vi "登陆界面.vi"() -> ()   [LabVIEW 2014]
panel:
  in  "注册":bool
  in  "游客登陆":bool
  out "学号与姓名表路径":path
  out "tips":string
  in  "姓  名":string
  in  "学  号":string
  in  "退出":bool
  in  "登陆":bool
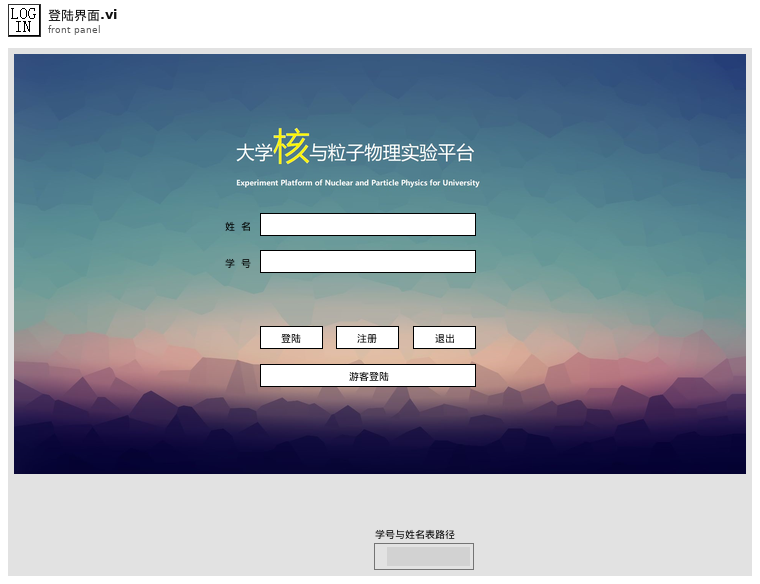
[diagram p1: front panel]
types:
  T1 = typedef "枚举常量_登陆界面.ctl" = enum16{"初始化", "等待用户输入", "信息匹配", "退出"}
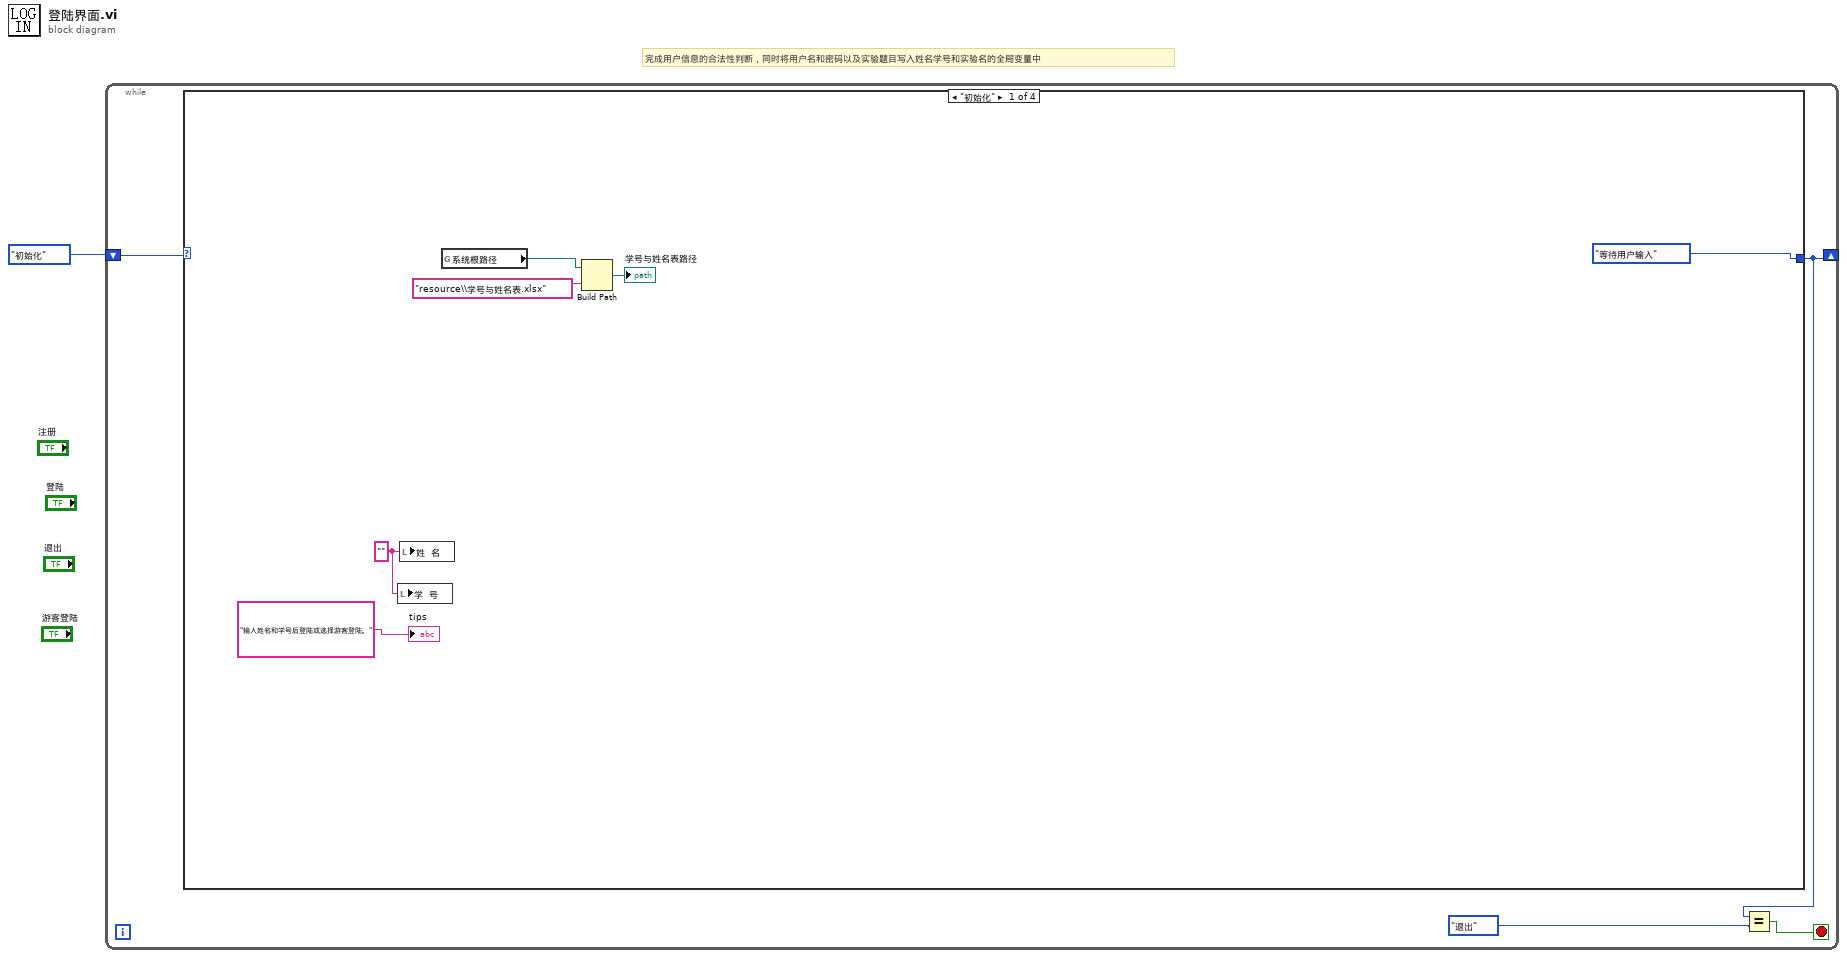
[diagram p0: block diagram]
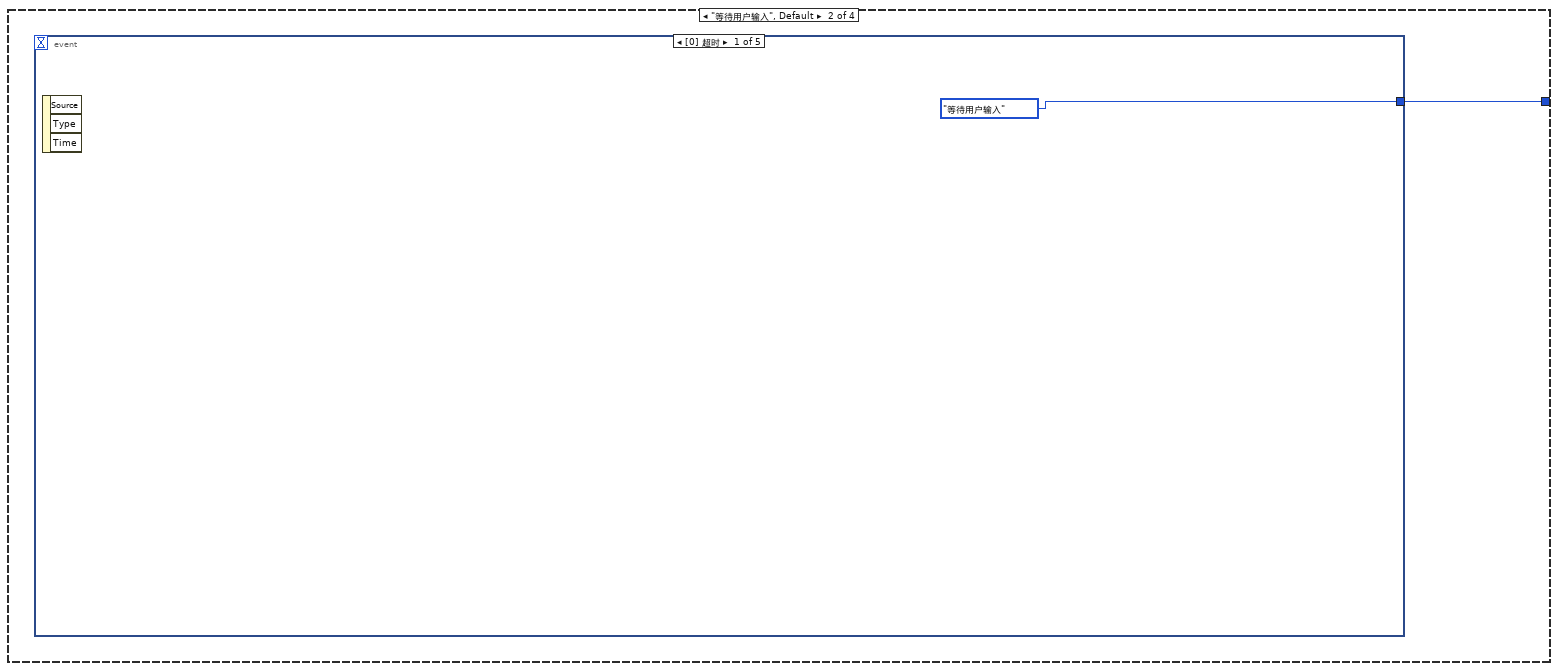
[diagram p2: hidden frame]
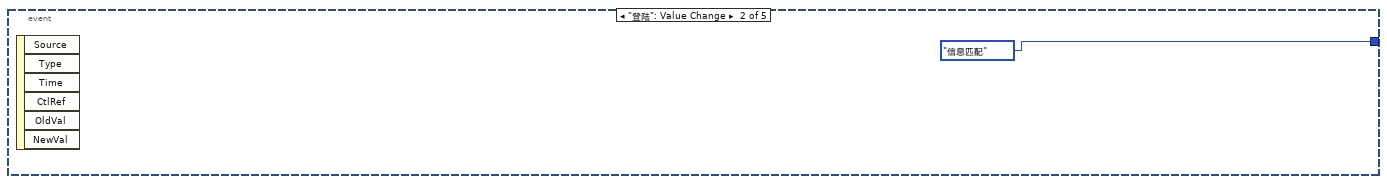
[diagram p3: hidden frame]
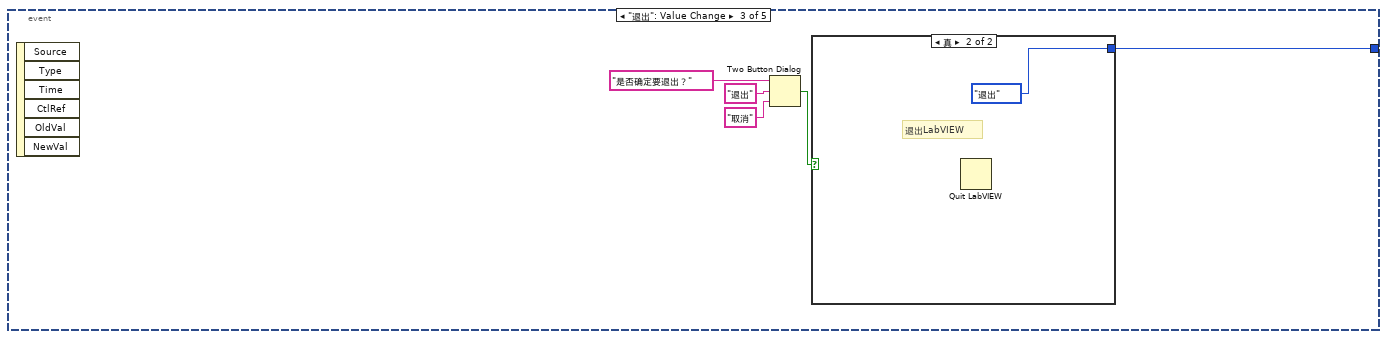
[diagram p4: hidden frame]
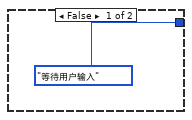
[diagram p5: hidden frame]
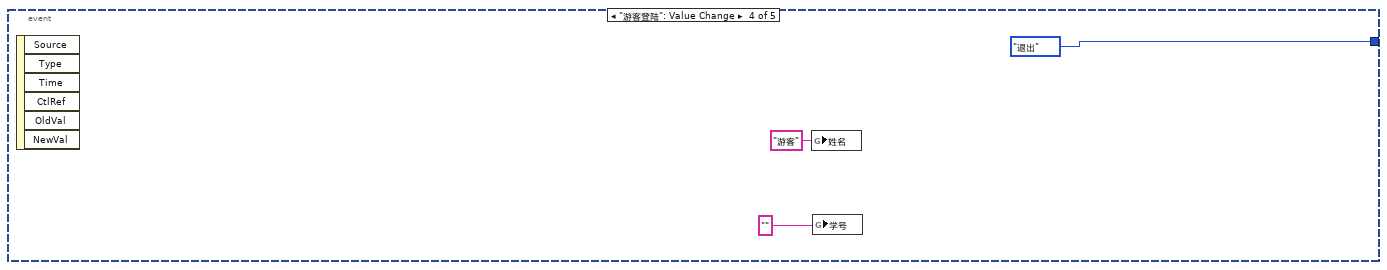
[diagram p6: hidden frame]
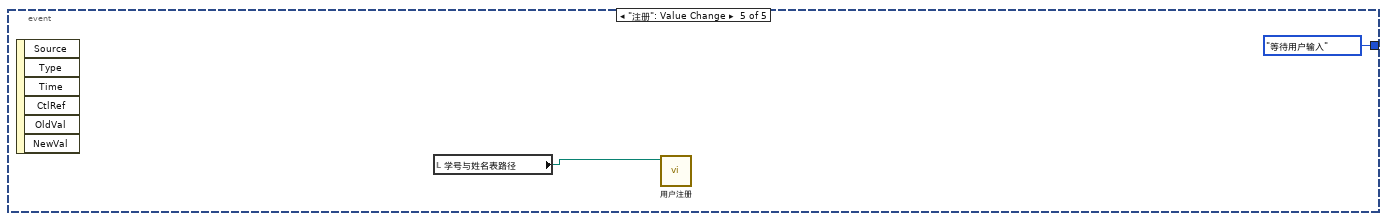
[diagram p7: hidden frame]
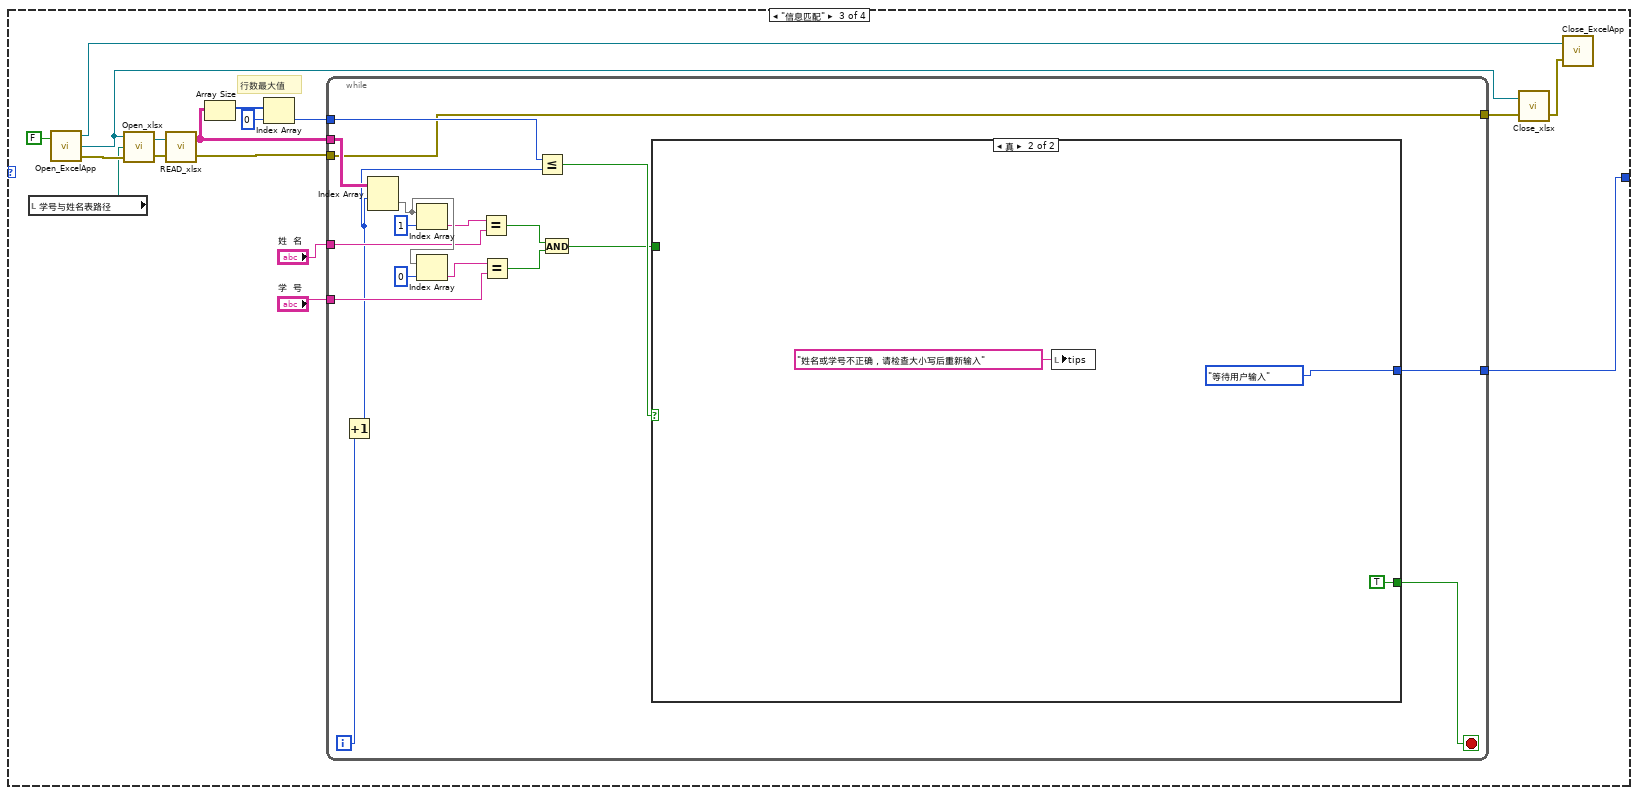
[diagram p8: hidden frame]
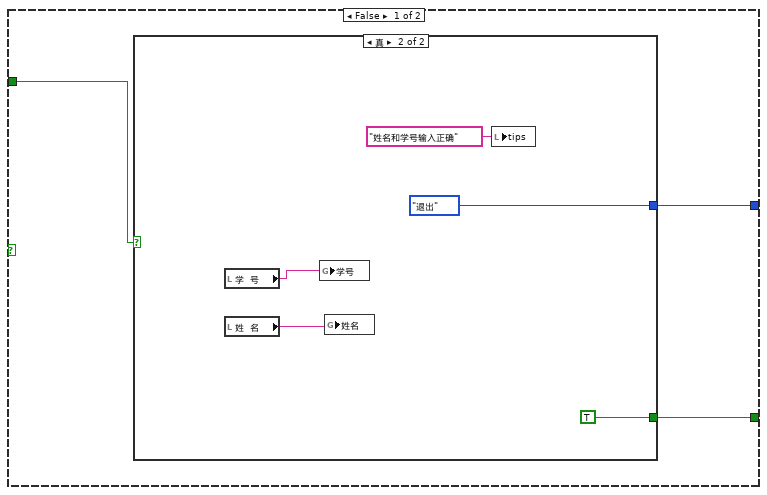
[diagram p9: hidden frame]
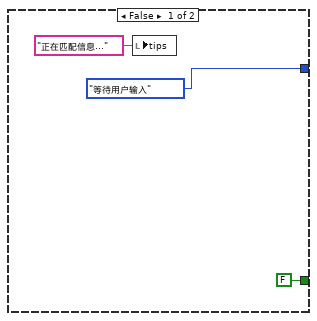
[diagram p10: hidden frame]
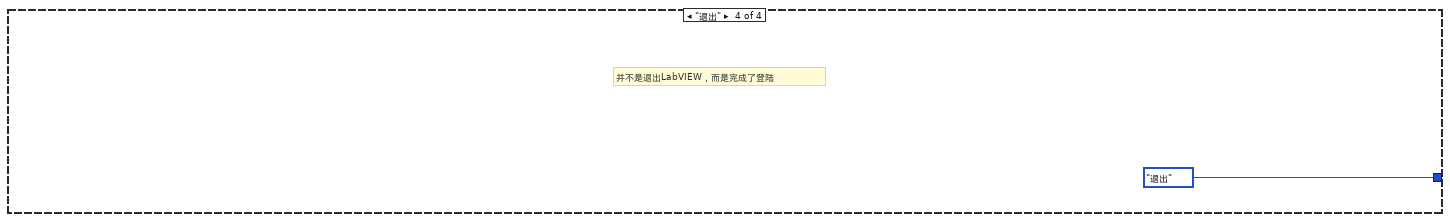
[diagram p11: hidden frame]
diagram:
  # "完成用户信息的合法性判断，同时将用户名和密码以及实验题目写入姓名学号和实验名的全局变量中"
  n1 = while {
    shift-right: [w2] -> _
    shift-left: 枚举常量_登陆界面."初始化" -> [w3]
    stop <- w4 stop-if-true
    n2 = case shown="\"初始化\"" w3 {
      tunnel: [枚举常量_登陆界面."等待用户输入" ("枚举") w12 w31 枚举常量_登陆界面."退出" ("枚举")] -> w2
      frame "初始化" {
        w11 = "" ("用户名")
        n3 = local write "学  号"(w11) -> ()
        n4 = local write "姓  名"(w11) -> ()
        n5 = global read "系统全局变量.vi" "系统根路径"() -> (w9:path)
        n6 = Build Path(base path=w9, name or relative path="resource\\学号与姓名表.xlsx" ("名称或相对路径")) -> (appended path=→"学号与姓名表路径":path)
        "tips" <- "输入姓名和学号后登陆或选择游客登陆。"
      }
      frame "等待用户输入", Default {
        n7 = event shown="[0] 超时" {
          selector: _ -> [_ _ _ _ _]
          dyn-events: _ -> [_ _ _ _ _]
          timeout: _ -> [_ _ _ _ _]
          tunnel: [枚举常量_登陆界面."等待用户输入" 枚举常量_登陆界面."信息匹配" w15 枚举常量_登陆界面."退出" 枚举常量_登陆界面."等待用户输入"] -> w12
          event Timeout {
            n8 = event-data() -> ()  [unwired: 1 in, 3 out]
          }
          event "登陆": Value Change {
            n9 = event-data() -> ()  [unwired: 1 in, 6 out]
          }
          event "退出": Value Change {
            n10 = event-data() -> ()  [unwired: 1 in, 6 out]
            n11 = Two Button Dialog(message="是否确定要退出？" ("消息"), 1:"取消" ("F按钮名称（“取消”）"), 2:"退出" ("T按钮名称（“确定”）")) -> (T button?=w16:bool)
            n12 = case shown="真" w16 {
              tunnel: [枚举常量_登陆界面."等待用户输入" 枚举常量_登陆界面."退出"] -> w15
              frame False {
              }
              frame True {
                # "退出LabVIEW"
                n13 = Quit LabVIEW() -> ()  [unwired: 1 in]
              }
            }
          }
          event "游客登陆": Value Change {
            n14 = event-data() -> ()  [unwired: 1 in, 6 out]
            n15 = global write "系统全局变量.vi" "姓名"("游客" ("姓名")) -> ()
            n16 = global write "系统全局变量.vi" "学号"("") -> ()
          }
          event "注册": Value Change {
            n17 = event-data() -> ()  [unwired: 1 in, 6 out]
            n18 = local read "学号与姓名表路径"() -> (w25:path)
            n19 = call "用户注册.vi"("excel路径"=w25) -> ()  [unwired: 10 in, 1 out]
          }
        }
      }
      frame "信息匹配" {
        # "行数最大值"
        n20 = local read "学号与姓名表路径"() -> (w41:path)
        n21 = call "Open_ExcelApp.vi"("excel是否可见"=FALSE) -> ("application引用"=w28:refnum<k7>, "documentl引用"=w29:refnum<k7>, "错误输出"=w42:errorcluster)  [unwired: 1 in]
        n22 = call "Open_xlsx.vi"("错误输入（无错误）"=w42, "excel路径"=w41, "document引用"=w29) -> ("错误输出"=w39:errorcluster, "该文档引用输出"=w40:refnum<k7>)
        n23 = call "READ_xlsx.vi"("错误输入（无错误）"=w39, "该文档引用输入"=w40) -> ("错误输出"=w38:errorcluster, "文档内容输出"=w35:string[][])
        n24 = Array Size(array=w35) -> (size(s)=w34:i32[])
        n25 = Index Array(array=w34, index=0 ("索引")) -> (element=w32:i32)
        n26 = while {
          tunnel: w35 -> [w51]
          tunnel: w38 -> [w44]
          tunnel: "姓  名" -> [w56]
          tunnel: "学  号" -> [w54]
          tunnel: w32 -> [w49]
          tunnel: [w45] -> w31
          tunnel: [w44] -> w27
          i -> [w61]
          stop <- w46 stop-if-true
          n27 = Increment(x=w61) -> (x+1=w50:i32)
          n28 = Index Array(array=w51, index (row)=w50) -> (element=w58:string[])  [unwired: 1 in]
          n29 = Index Array(array=w58, index=1 ("索引")) -> (element=w57:string)
          n30 = Index Array(array=w58, index=0 ("索引")) -> (element=w55:string)
          n31 = Equal?(x=w57, y=w56) -> (x = y?=w53:bool)
          n32 = Equal?(x=w55, y=w54) -> (x = y?=w52:bool)
          n33 = Less Or Equal?(x=w49, y=w50) -> (x <= y?=w48:bool)
          n34 = And(x=w53, y=w52) -> (x .and. y?=w47:bool)
          n35 = case shown="真" w48 {
            tunnel: w47 -> [w64 _]
            tunnel: [w63 TRUE] -> w46
            tunnel: [w62 枚举常量_登陆界面."等待用户输入"] -> w45
            frame False {
              n36 = case shown="真" w64 {
                tunnel: [FALSE TRUE] -> w63
                tunnel: [枚举常量_登陆界面."等待用户输入" 枚举常量_登陆界面."退出"] -> w62
                frame False {
                  n37 = local write "tips"("正在匹配信息..." ("tips")) -> ()
                }
                frame True {
                  n38 = local read "学  号"() -> (w69:string)
                  n39 = local read "姓  名"() -> (w68:string)
                  n40 = global write "系统全局变量.vi" "学号"(w69) -> ()
                  n41 = global write "系统全局变量.vi" "姓名"(w68) -> ()
                  n42 = local write "tips"("姓名和学号输入正确" ("tips")) -> ()
                }
              }
            }
            frame True {
              n43 = local write "tips"("姓名或学号不正确，请检查大小写后重新输入" ("tips")) -> ()
            }
          }
        }
        n44 = call "Close_xlsx.vi"("错误输入（无错误）"=w27, "document引用"=w29) -> ("错误输出"=w30:errorcluster)  [unwired: 1 in]
        n45 = call "Close_ExcelApp.vi"("错误输入（无错误）"=w30, "application引用"=w28) -> ()  [unwired: 1 in, 1 out]
      }
      frame "退出" {
        # "并不是退出LabVIEW，而是完成了登陆"
      }
    }
    n46 = Equal?(x=w2, y=枚举常量_登陆界面."退出" ("枚举")) -> (x = y?=w4:bool)
  }
